vi "h.NET.GetStaticNetworkSettings.vi"(5 "error in":errorcluster, 6 "Connection ID":refnum<k5>) -> (0 "error out":errorcluster, 1 "Netmask":string, 2 "IP Address":string, 3 "Connection ID":refnum<k5>, 4 "Gateway":string)   [LabVIEW 2016, in "h.Library.lvlib"]
doc: "This vi retrieves the static network settings. These are the settings that take affect when the network mode is set to static.\n\n<b>Connection ID</b> - is a network connection refnum that uniquely identifies the TCP connection\n<b>error in</b> - describes error conditions that occur before this node runs. This input provides standard error functionality\n<b>Connection ID out</b> - returns the same value as connection ID\n<b>IP Address</b> - static IP address\n<b>Netmask</b> - static Netmask\n<b>Gateway</b> - statics Gateway\n<b>error out</b> - contains error information. This output provides standard error out functionality."
uses:
  h.Library.lvlib
panel:
  out "Message":string
  # "Hyperion Get Static Network Settings"
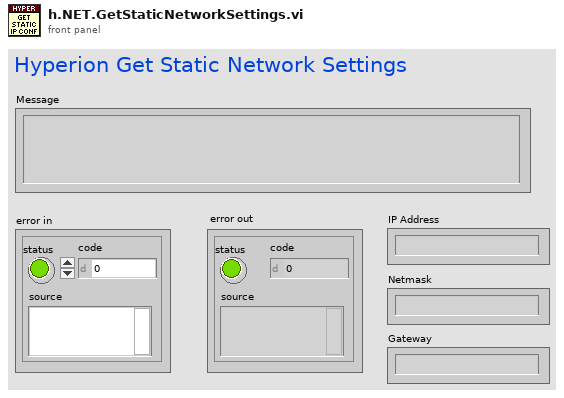
[diagram p1: front panel]
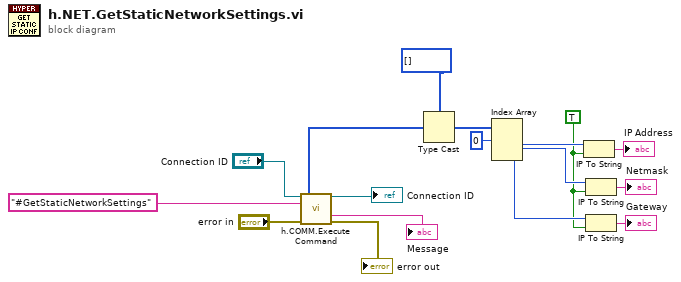
[diagram p0: block diagram]
diagram:
  w1 = TRUE ("dot notation? (F)")
  n1 = call "h.COMM.Execute Command.vi"("Connection ID"="Connection ID", "Command"="#GetStaticNetworkSettings", "error in"="error in") -> ("Content"=w10:u8[], "Connection ID out"=→"Connection ID":refnum<k5>, "Message"=→"Message":string, "error out"=→"error out":errorcluster)  [unwired: 5 in, 4 out]
  n2 = Type Cast(type=u32[] [], x=w10) -> (*(type *) &x=w9:u32[])
  n3 = Index Array(array=w9, index #1=0 ("index")) -> (element #1=w7:u32, element #2=w3:u32, element #3=w2:u32)  [unwired: 2 in]
  n4 = IP To String(1:w1, 2:w7) -> (0:→"IP Address":string)
  n5 = IP To String(1:w1, 2:w3) -> (0:→"Netmask":string)
  n6 = IP To String(1:w1, 2:w2) -> (0:→"Gateway":string)
